vi "fpga rw tester.vi"() -> ()   [LabVIEW 2013]
uses:
  <vilib>/userdefined/High Color/nirio_resource_hc.ctl
  <vilib>/FPGAPlugInAG/PCIe-7852R/niLvFpga_Open_PCIe-7852R.vi
  <vilib>/rvi/interface/common/niFpgaWaitOnOcc.vi
  <vilib>/Utility/error.llb/Error Cluster From Error Code.vi
  <vilib>/rvi/errors/niLvFpgaAdjustHostInterfaceError.vi
  <vilib>/rvi/interface/nirviOpenFPGA/nirviOpenFPGA.xnode
  openfpgaref.8.6.ctl
  FPGA Bitfiles/UHR-FleezersInst_FPGATarget_UHR-Fleezers_Leonardo042018V4.lvbitx
  <vilib>/rvi/interface/nirviMethod/nirviMethod.xnode
  <vilib>/rvi/errors/niLvFpgaMergeErrorWithErrorCode.vi
  <vilib>/FPGAPlugInAG/PCIe-7852R/niLvFpga_ReadFifo_PCIe-7852R.vi
panel:
  out "error out":errorcluster
  out "Data qpd":i16[](array[numeric])
  out "Data pos":u16[](array[numeric])
  in  "Numeric":dbl
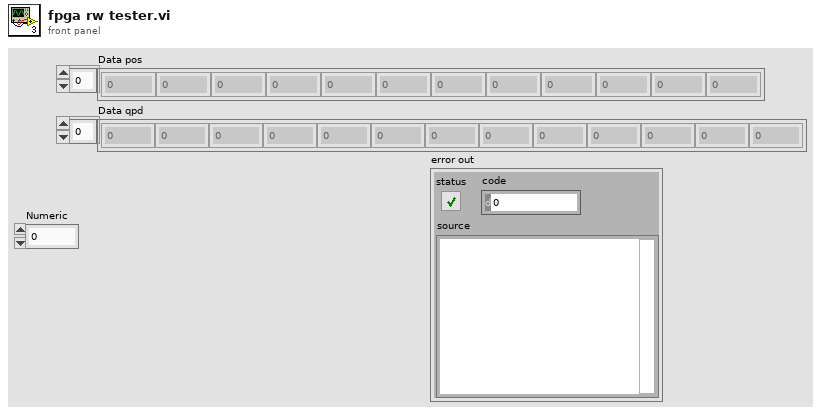
[diagram p1: front panel]
types:
  T1 = typedef "nirio_resource_hc.ctl" = tag
  T2 = typedef "openfpgaref.8.6.ctl" = refnum<k20>
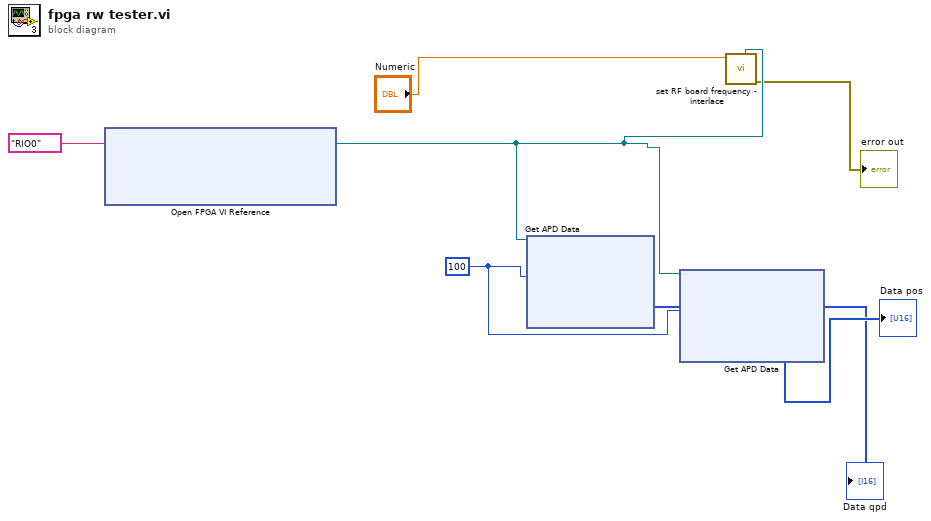
[diagram p0: block diagram]
diagram:
  w6 = u32 100 ("Number of Elements")
  n1 = xnode "Open FPGA VI Reference"("resource name"=T1 "RIO0") -> ("FPGA VI Reference Out"=w2:T2)  [unwired: 1 in, 1 out]
  n2 = xnode "Get APD Data"("FPGA VI Reference In"=w2, "Number of Elements"=w6) -> ("Data"=→"Data qpd":i16[])  [unwired: 2 in, 3 out]
  n3 = xnode "Get APD Data"("FPGA VI Reference In"=w2, "Number of Elements"=w6) -> ("Data"=→"Data pos":u16[])  [unwired: 2 in, 3 out]
  n4 = call "set RF board frequency - interlace.vi"("FPGA VI Reference In"=w2, "Board 1 Frequency 1  (MHz)"="Numeric") -> ("error out"=→"error out":errorcluster)  [unwired: 8 in, 1 out]
